vi "to string.vi"(8 "error in":errorcluster, 11 "fixed channel configuration in":refnum<class "fixed channel configuration.lvclass">) -> (0 "error out":errorcluster, 1 "data":string, 2 "version":string, 3 "fixed channel configuration out":refnum<class "fixed channel configuration.lvclass">)   [LabVIEW 2013, in "fixed channel configuration.lvclass"]
doc: "Provides an interface for saving a module configuration to a file or other serialized data source. It is recommended that all children of this class store data in two sets--data required for its own initialization, and any data required for parent initialization--and that each implementation uses the <b>Call Parent Method</b> primitive to serialize parent information.\nNI Tag Bus Module Framework 1.0.3.43\nNI Systems Engineering"
uses:
  fixed channel configuration.lvclass
  <vilib>/NI/Tag Bus Module Framework/module configuration/TBM module configuration.lvclass
  <vilib>/NI/Tag Bus Module Framework/channel/TBM channel.lvclass
  <vilib>/NI/Configuration Framework/serializable configuration/NISE_CEF_serializable configuration.lvclass
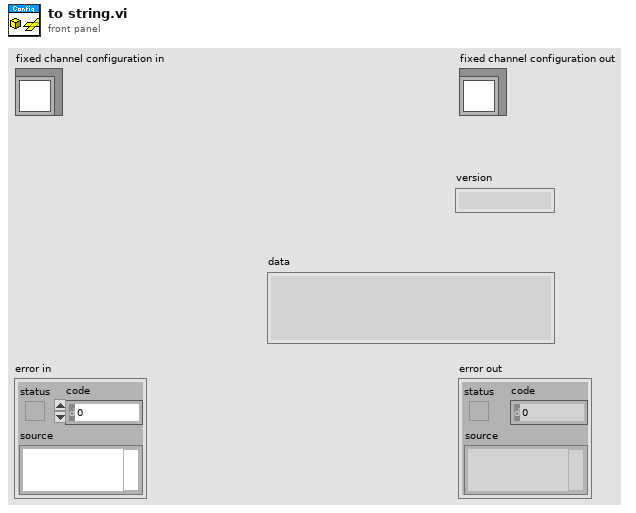
[diagram p1: front panel]
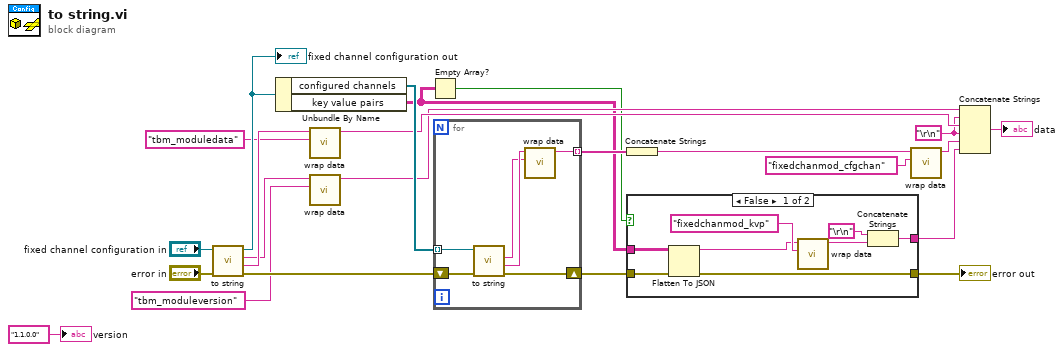
[diagram p0: block diagram]
diagram:
  w5 = "\r\n"
  n1 = call-parent "to string.vi"("error in"="error in", "module configuration in"="fixed channel configuration in") -> ("error out"=w19:errorcluster, "data"=w10:string, "version"=w9:string, "module configuration out"=w21:refnum<class "fixed channel configuration.lvclass">)  [unwired: 6 in]
  "fixed channel configuration out" <- w21
  n2 = Unbundle By Name(w21) -> ("configured channels"=w18:refnum<class "TBM channel.lvclass">[], "key value pairs"=w3:string[][])
  n3 = call <vilib>:"wrap data.vi"("identifier"="tbm_moduledata", "data to wrap"=w10) -> ("wrapped data"=w12:string)  [unwired: 9 in]
  n4 = call <vilib>:"wrap data.vi"("identifier"="tbm_moduleversion", "data to wrap"=w9) -> ("wrapped data"=w11:string)  [unwired: 9 in]
  n5 = Empty Array?(array=w3) -> (empty?=w4:bool)
  n6 = for {
    tunnel: w18 -> [w29] mode=indexing
    shift-right: [w25] -> w2
    shift-left: w19 -> [w26]
    tunnel: [w24] -> w14 mode=indexing
    n7 = call-dynamic "to string.vi"("error in"=w26, "channel in"=w29) -> ("error out"=w25:errorcluster, "channel data"=w28:string, "identifier"=w27:string)  [unwired: 6 in, 1 out]
    n8 = call <vilib>:"wrap data.vi"("identifier"=w27, "data to wrap"=w28) -> ("wrapped data"=w24:string)  [unwired: 9 in]
  }
  n9 = Concatenate Strings(w14) -> (w13:string)
  n10 = case shown="False" w4 {
    tunnel: [w35 _] -> w6
    tunnel: w3 -> [w32 _]
    tunnel: w2 -> [w33 w38]
    tunnel: [w30 w38] -> w1
    frame False {
      n11 = Flatten To JSON(anything=w32, error in (no error)=w33) -> (JSON string=w31:string, 11:w30:errorcluster)  [unwired: 1 in]
      n12 = call <vilib>:"wrap data.vi"("identifier"="fixedchanmod_kvp", "data to wrap"=w31) -> ("wrapped data"=w36:string)  [unwired: 9 in]
      n13 = Concatenate Strings("\r\n", w36) -> (w35:string)
    }
    frame True {
    }
  }
  "error out" <- w1
  n14 = call <vilib>:"wrap data.vi"("identifier"="fixedchanmod_cfgchan", "data to wrap"=w13) -> ("wrapped data"=w17:string)  [unwired: 9 in]
  n15 = Concatenate Strings(w11, w5, w12, w5, w17, w6) -> (→"data":string)
  "version" <- "1.1.0.0" ("version")
